vi "WristButton.vi"(11 "ClusterIN":T1) -> (1 "Angle Out":dbl format="%#_13g")   [LabVIEW 2018]
uses:
  TypeDefs/Teleop Data Cluster.ctl
  TypeDefs/Joystick Buttons.ctl
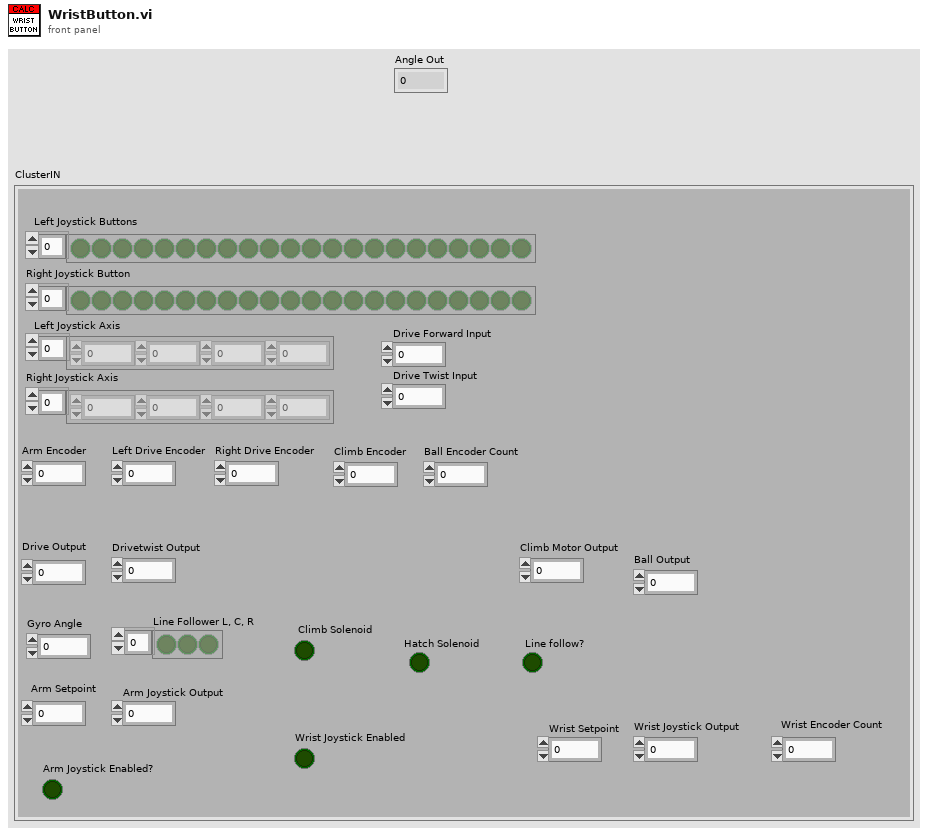
[diagram p1: front panel]
types:
  T1 = typedef "Teleop Data Cluster.ctl" = cluster{"Drive Forward Input ":dbl, "Drive Twist Input":dbl, "Drive Output":dbl, "Drivetwist Output":dbl, "Left Joystick Buttons":bool[], "Left Joystick Axis":dbl[], "Right Joystick Axis":dbl[], "Right Joystick Button":bool[], "Arm Encoder":dbl, "Left Drive Encoder":dbl, "Right Drive Encoder":dbl, "Gyro Angle ":dbl, "Arm Joystick Output  ":dbl, "Line Follower L, C, R ":bool[], "Line follow?":bool, " Climb Solenoid":bool, "Wrist Encoder Count":dbl, "Wrist Joystick Output":dbl, "Ball Encoder Count":dbl, "Ball Output":dbl, "Climb Encoder":dbl, "Climb Motor Output":dbl, " Hatch Solenoid":bool, "Arm Setpoint ":dbl, "Wrist Setpoint ":dbl, "Arm Joystick Enabled?":bool, "Wrist Joystick Enabled":bool}
  T2 = typedef "Joystick Buttons.ctl" = enum16{"Trigger", "Thumb", "Top 3", "Top 4", "Top 5", "Top 6", "Bottom 7", "Bottom 8", "Bottom 9", "Bottom 10", "Bottom 11", "Bottom 12"}
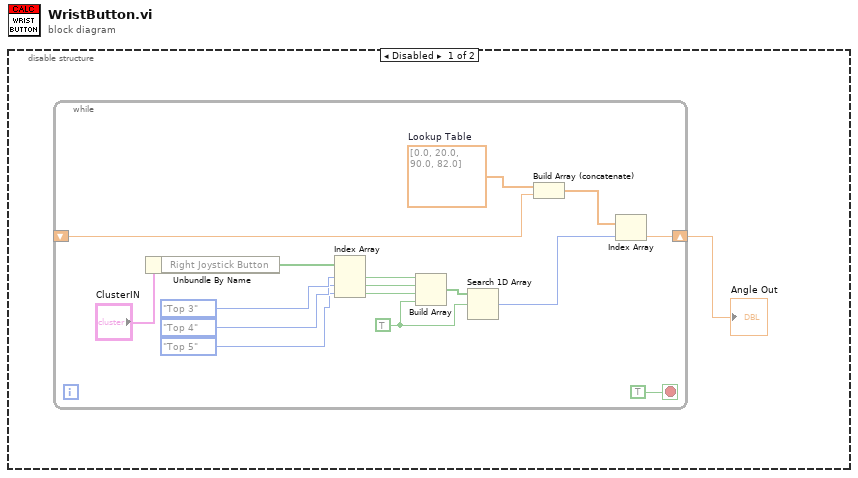
[diagram p0: block diagram]
diagram:
  n1 = disable-structure shown="Disabled" {
    frame Disabled {
      n2 = while {
        shift-right: [w8] -> w1
        shift-left: _ -> [w6]
        stop <- TRUE stop-if-true
        w10 = dbl[] [0.0, 20.0, 90.0, 82.0]  # Lookup Table
        w2 = TRUE ("element")
        n3 = Unbundle By Name("ClusterIN") -> ("Right Joystick Button"=w16:bool[])
        n4 = Index Array(array=w16, index #1=Joystick_Buttons."Top 3" ("Enum"), index #2=Joystick_Buttons."Top 4" ("Enum"), index #3=Joystick_Buttons."Top 5" ("Enum")) -> (element #1=w15:bool, element #2=w14:bool, element #3=w13:bool)
        n5 = Build Array(w15, w14, w13, w2) -> (w12:bool[])
        n6 = Search 1D Array(1D array=w12, element=w2) -> (index of element=w11:i32)  [unwired: 1 in]
        n7 = Build Array (concatenate)(w10, w6) -> (w7:dbl[])
        n8 = Index Array(array=w7, index=w11) -> (element=w8:dbl)
      }
      "Angle Out" <- w1
    }
    frame Enabled {
    }
  }
